vi "HO4.vi"(3 "?":bool, 4 "Delay (ms)":i16=500, 5 "Min":dbl=100.0, 6 "Max":dbl=500.0) -> (0 "Sweep Chart":dbl(graph), 1 "Scope Chart":dbl(graph), 2 "Strip Chart":cluster{"Double":dbl, dbl, "Max":dbl, "Min":dbl}(graph))   [LabVIEW 2020]
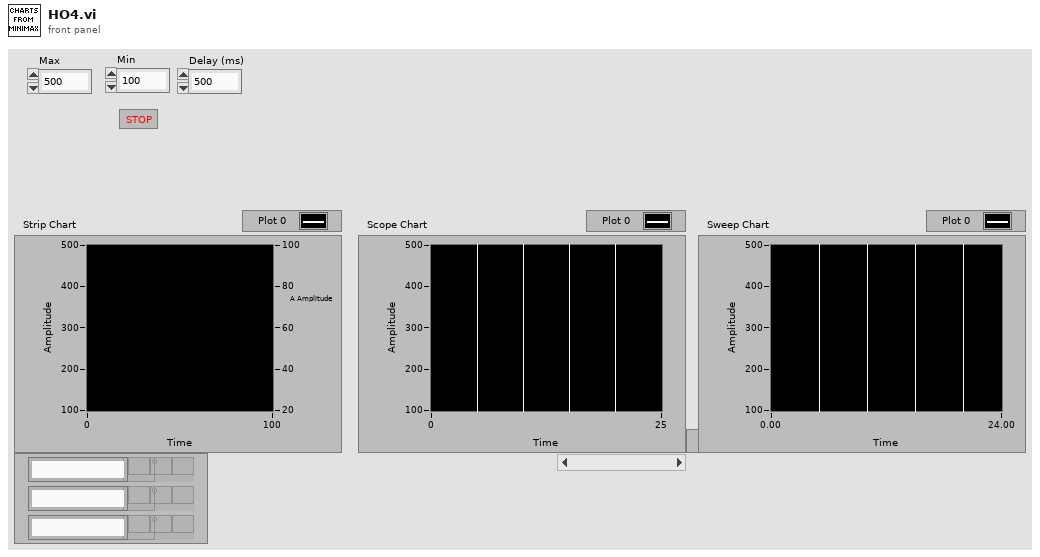
[diagram p1: front panel]
types:
  T1 = cluster{"Double":dbl, dbl, "Max":dbl, "Min":dbl}[]
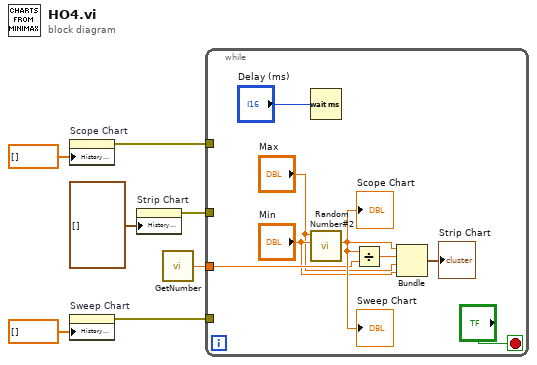
[diagram p0: block diagram]
diagram:
  n1 = property on="Scope Chart" class="WFChart (strict)"("History Data"=dbl[] []) -> (error out=w5:errorcluster)  [unwired: 2 in, 1 out]
  n2 = property on="Sweep Chart" class="WFChart (strict)"("History Data"=dbl[] []) -> (error out=w6:errorcluster)  [unwired: 2 in, 1 out]
  n3 = property on="Strip Chart" class="WFChart (strict)"("History Data"=T1 []) -> (error out=w7:errorcluster)  [unwired: 2 in, 1 out]
  n4 = call "GetNumber.vi"() -> ("Numeric"=w1:dbl)
  n5 = while {
    tunnel: w7 -> [_]
    tunnel: w6 -> [_]
    tunnel: w5 -> [_]
    tunnel: w1 -> [w10]
    stop <- "?" stop-if-true
    n6 = Wait (ms)(milliseconds to wait="Delay (ms)") -> ()  [unwired: 1 out]
    n7 = call "Random Number#2.vi"("Maximum"="Max", "Minimum"="Min") -> ("Double"=w11:dbl)  [unwired: 4 in, 3 out]
    "Scope Chart" <- w11
    "Sweep Chart" <- w11
    n8 = Divide(x=w11, y=w10) -> (x/y=w12:dbl)
    n9 = Bundle("Double"=w11, w12, "Max"="Max", "Min"="Min") -> (→"Strip Chart":cluster{"Double":dbl, dbl, "Max":dbl, "Min":dbl})  [unwired: 1 in]
  }
